vi "PixieGetData.vi"(8 "error IO":errorcluster) -> (0 "error out":errorcluster, 1 "PixieTimes":T1, 2 "Histogram Data":u32[][](array[numeric]))   [LabVIEW 2013]
uses:
  ctl/PixieTimes.ctl
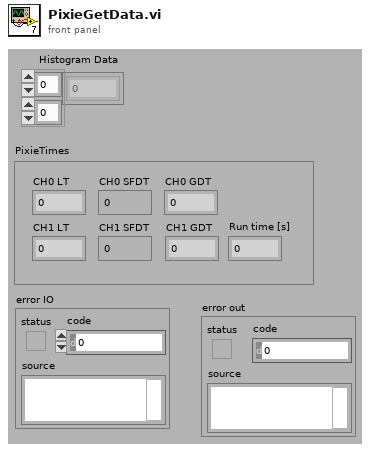
[diagram p1: front panel]
types:
  T1 = typedef "PixieTimes.ctl" = cluster{"CH0 LT":dbl, "CH1 LT":dbl, "CH0 SFDT":dbl, "CH1 SFDT":dbl, "CH0 GDT":dbl, "CH1 GDT":dbl, "Run time [s]":dbl}
  T2 = cluster{"livetime":dbl, "livetime":dbl, "SFDT":dbl, "SFDT":dbl, "GDT":dbl, "GDT":dbl, "Run time [s]":dbl}
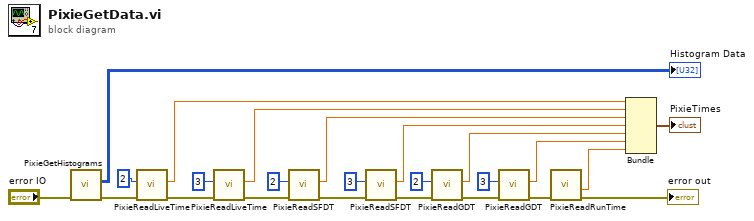
[diagram p0: block diagram]
diagram:
  n1 = call "PixieGetHistograms.vi"("error in (no error)"="error IO") -> ("error out"=w1:errorcluster, "Histogram Data"=→"Histogram Data":u32[][])  [unwired: 1 in, 8 out]
  n2 = call "PixieReadLiveTime.vi"("error in (no error)"=w1, "ChanNum"=u16 2) -> ("error out"=w24:errorcluster, "livetime"=w11:dbl)  [unwired: 8 out]
  n3 = call "PixieReadLiveTime.vi"("error in (no error)"=w24, "ChanNum"=u16 3) -> ("error out"=w20:errorcluster, "livetime"=w10:dbl)  [unwired: 8 out]
  n4 = call "PixieReadSFDT.vi"("error in (no error)"=w20, "ChanNum"=u16 2) -> ("error out"=w17:errorcluster, "SFDT"=w9:dbl)  [unwired: 8 in]
  n5 = call "PixieReadSFDT.vi"("error in (no error)"=w17, "ChanNum"=u16 3) -> ("error out"=w15:errorcluster, "SFDT"=w8:dbl)  [unwired: 8 in]
  n6 = call "PixieReadGDT.vi"("error in (no error)"=w15, "ChanNum"=u16 2) -> ("error out"=w16:errorcluster, "GDT"=w7:dbl)  [unwired: 8 in]
  n7 = call "PixieReadGDT.vi"("error in (no error)"=w16, "ChanNum"=u16 3) -> ("error out"=w14:errorcluster, "GDT"=w6:dbl)  [unwired: 8 in]
  n8 = call "PixieReadRunTime.vi"("error in (no error)"=w14) -> ("error out"=→"error out":errorcluster, "Run time [s]"=w5:dbl)  [unwired: 1 in, 8 out]
  n9 = Bundle("livetime"=w11, "livetime"=w10, "SFDT"=w9, "SFDT"=w8, "GDT"=w7, "GDT"=w6, "Run time [s]"=w5) -> (→"PixieTimes":T2)  [unwired: 1 in]
